vi "SDG60ConfTrigger.vi"(0 "VISA resource name":refnum<visa-resource-name>="USB0::0xF4EC::0x1101::SDG6XEBC5R0119::INSTR", 4 "Burst Delay (1.352 us)":dbl=1.352e-06, 5 "error in (no error)":errorcluster, 6 "Trigger Source (0: Internal)":u16(ring) items=["Internal", "External", "Manual"], 7 "External Trigger Condition (0: Rise)":u16(ring) items=["Rise", "Fall"], 8 "Enable Burst Mode (T:Enable)":bool=TRUE, 10 "Channel (1:Channel 1)":i32(ring)=1 items=["Channel 1"=1, "Channel 2"=2], 11 "Trigger Out Mode (0: Off)":u16(ring) items=["Off", "Rise", "Fall"]) -> (14 "VISA resource name out":refnum<visa-resource-name>, 19 "error out":errorcluster)   [LabVIEW 2018]
doc: "Configures and enables burst output mode.\n\nNote: Burst mode is not available for noise waveform."
panel:
  in  "Burst Period (0.01 s)":dbl=0.01 format="%#.3g"
  # "Trigger enables through burst mode"
  # "Trigger High: 2-5.5V\nTrigger Low: -0.5-0.8V"
  # "Range: 1.352us-100s"
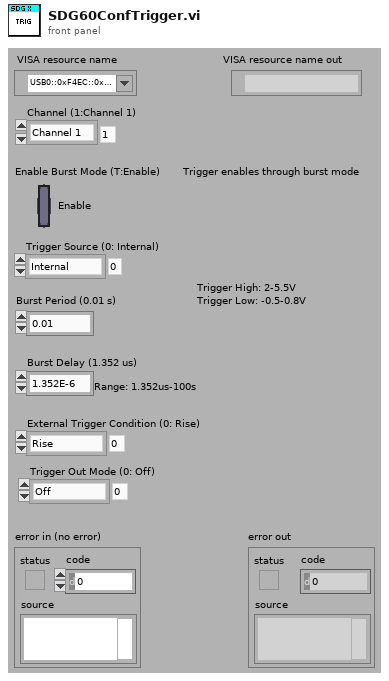
[diagram p1: front panel]
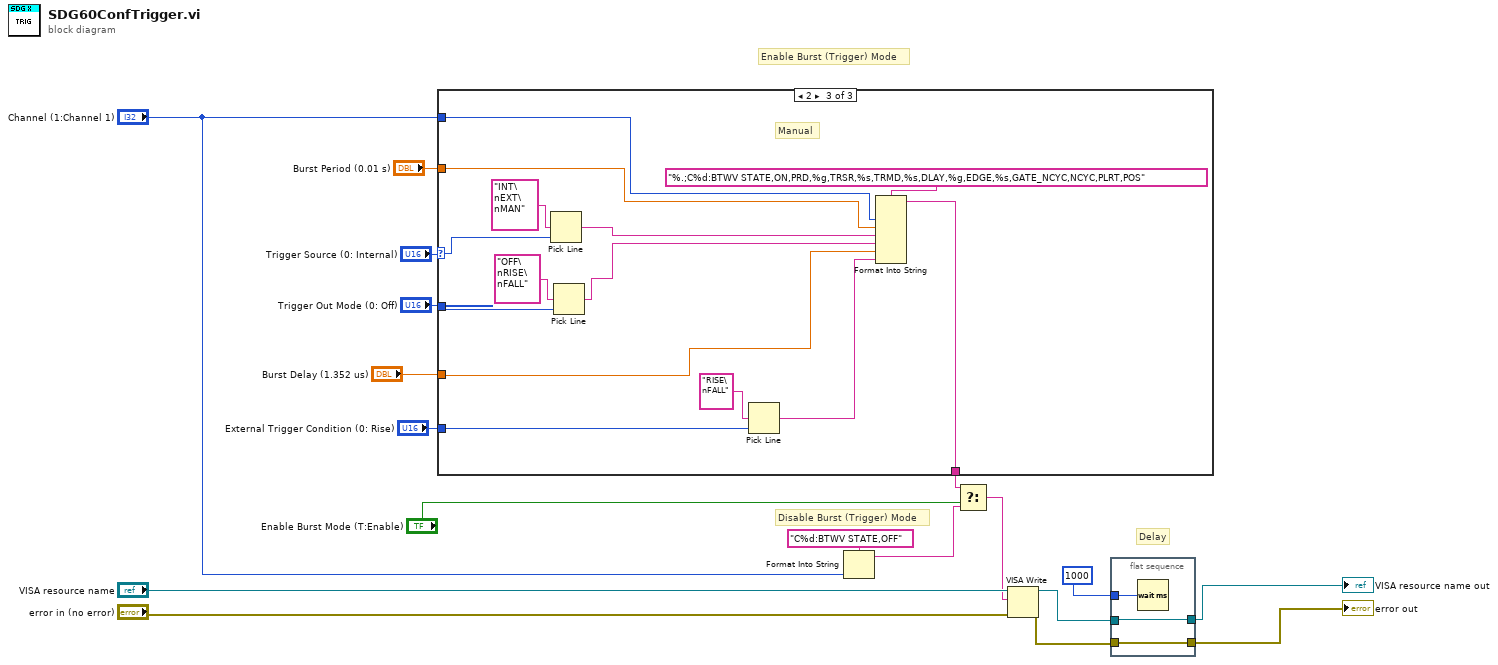
[diagram p0: block diagram]
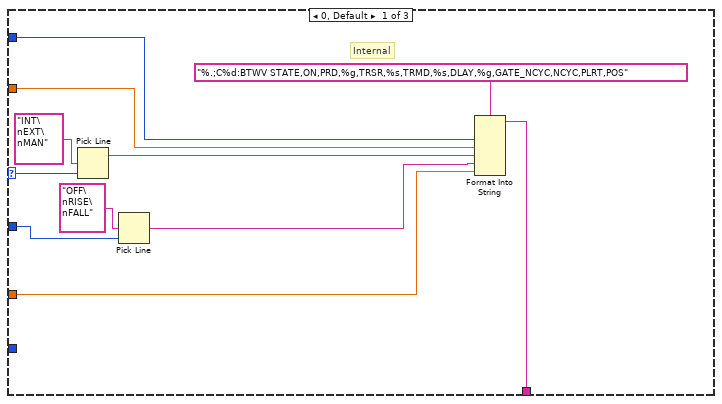
[diagram p2: hidden frame]
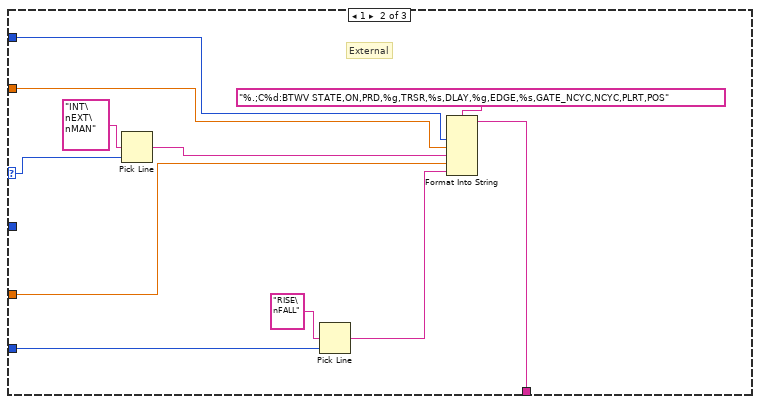
[diagram p3: hidden frame]
diagram:
  # "Delay"
  # "Disable Burst (Trigger) Mode"
  # "Enable Burst (Trigger) Mode"
  n1 = case shown="2" "Trigger Source (0: Internal)" {
    selector: "Trigger Source (0: Internal)" -> [w26 w34 w49]
    tunnel: "Channel (1:Channel 1)" -> [w27 w33 w48]
    tunnel: "Burst Delay (1.352 us)" -> [w21 w30 w43]
    tunnel: [w19 w31 w46] -> w12
    tunnel: "Trigger Out Mode (0: Off)" -> [w20 _ w44]
    tunnel: "External Trigger Condition (0: Rise)" -> [_ w35 w50]
    tunnel: "Burst Period (0.01 s)" -> [w24 w32 w47]
    frame 0, Default {
      # "Internal"
      n2 = Pick Line(multi-line string="INT\nEXT\nMAN", line index=w26) -> (output string=w23:string)  [unwired: 1 in]
      n3 = Pick Line(multi-line string="OFF\nRISE\nFALL", line index=w20) -> (output string=w22:string)  [unwired: 1 in]
      n4 = Format Into String(format string="%.;C%d:BTWV STATE,ON,PRD,%g,TRSR,%s,TRMD,%s,DLAY,%g,GATE_NCYC,NCYC,PLRT,POS", w27, w24, w23, w22, w21) -> (resulting string=w19:string)  [unwired: 2 in, 1 out]
    }
    frame 1 {
      # "External"
      n5 = Pick Line(multi-line string="INT\nEXT\nMAN", line index=w34) -> (output string=w37:string)  [unwired: 1 in]
      n6 = Pick Line(multi-line string="RISE\nFALL", line index=w35) -> (output string=w36:string)  [unwired: 1 in]
      n7 = Format Into String(format string="%.;C%d:BTWV STATE,ON,PRD,%g,TRSR,%s,DLAY,%g,EDGE,%s,GATE_NCYC,NCYC,PLRT,POS", w33, w32, w37, w30, w36) -> (resulting string=w31:string)  [unwired: 2 in, 1 out]
    }
    frame 2 {
      # "Manual"
      n8 = Pick Line(multi-line string="INT\nEXT\nMAN", line index=w49) -> (output string=w51:string)  [unwired: 1 in]
      n9 = Pick Line(multi-line string="OFF\nRISE\nFALL", line index=w44) -> (output string=w41:string)  [unwired: 1 in]
      n10 = Pick Line(multi-line string="RISE\nFALL", line index=w50) -> (output string=w42:string)  [unwired: 1 in]
      n11 = Format Into String(format string="%.;C%d:BTWV STATE,ON,PRD,%g,TRSR,%s,TRMD,%s,DLAY,%g,EDGE,%s,GATE_NCYC,NCYC,PLRT,POS", w48, w47, w51, w41, w43, w42) -> (resulting string=w46:string)  [unwired: 2 in, 1 out]
    }
  }
  n12 = Format Into String(format string="C%d:BTWV STATE,OFF", "Channel (1:Channel 1)") -> (resulting string=w10:string)  [unwired: 2 in, 1 out]
  n13 = Select(t=w12, s="Enable Burst Mode (T:Enable)", f=w10) -> (s? t:f=w9:string)
  n14 = VISA Write(VISA resource name="VISA resource name", write buffer=w9, error in (no error)="error in (no error)") -> (VISA resource name out=w6:refnum<visa-resource-name>, error out=w4:errorcluster)  [unwired: 1 out]
  n15 = flat-sequence {
    tunnel: w4 -> [w57]
    tunnel: [w57] -> w2
    tunnel: u32 1000 ("Delay Time (10)") -> [w56]
    tunnel: w6 -> [w55]
    tunnel: [w55] -> w3
    frame #0 {
      n16 = Wait (ms)(milliseconds to wait=w56) -> ()  [unwired: 1 out]
    }
  }
  "error out" <- w2
  "VISA resource name out" <- w3
